vi "Simplex_FunctionValues_AE.vi"(0 "F(x) - Evaluation Results":dbl[](array[numeric]), 2 "Action":T1, 11 "x Values - Amount of Modes":dbl[][](array[numeric])) -> (4 "F(x) - Evaluation Results Out":dbl[](array[numeric]), 15 "x Values - Amount of Modes Out":dbl[][](array[numeric]))   [LabVIEW 2014]
uses:
  Standard Action.ctl
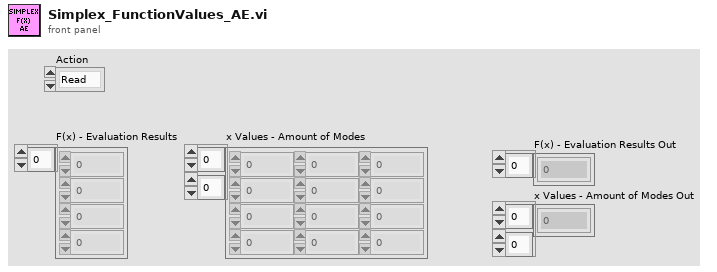
[diagram p1: front panel]
types:
  T1 = typedef "Standard Action.ctl" = enum16{"Read", "Write"}
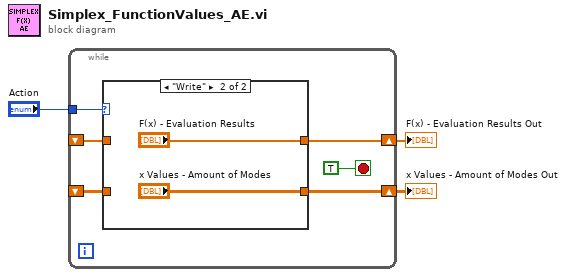
[diagram p0: block diagram]
diagram:
  n1 = while {
    shift-right: [w7] -> w2
    shift-left: _ -> [w5]
    shift-right: [w6] -> w1
    shift-left: _ -> [w4]
    tunnel: "Action" -> [w8]
    stop <- TRUE stop-if-true
    n2 = case shown="\"Write\"" w8 {
      tunnel: [w11 "F(x) - Evaluation Results"] -> w7
      tunnel: [w10 "x Values - Amount of Modes"] -> w6
      tunnel: w5 -> [w11 _]
      tunnel: w4 -> [w10 _]
      frame "Read", Default {
      }
      frame "Write" {
      }
    }
  }
  "F(x) - Evaluation Results Out" <- w2
  "x Values - Amount of Modes Out" <- w1
